vi "UI Event Handler.vi"() -> ()   [LabVIEW 2015]
panel:
  in  "Time Check":bool
  out "Iteration":i32
  in  "Stop":bool
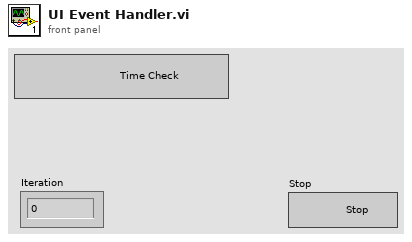
[diagram p1: front panel]
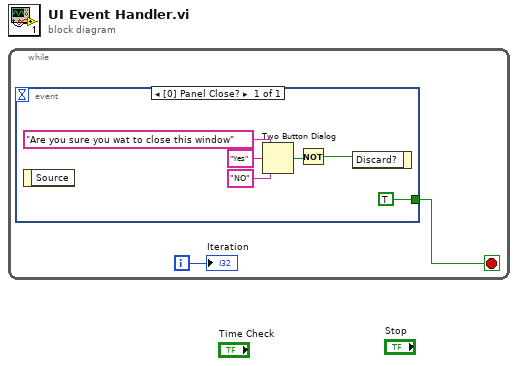
[diagram p0: block diagram]
diagram:
  n1 = while {
    i -> [w2]
    stop <- w1 stop-if-true
    n2 = event shown="[0] Panel Close?" {
      selector: _ -> [_]
      dyn-events: _ -> [_]
      timeout: _ -> [_]
      tunnel: [TRUE] -> w1
      event Panel Close? {
        n3 = event-data() -> ()  [unwired: 1 in, 1 out]
        n4 = Two Button Dialog(message="Are you sure you wat to close this window", 1:"NO" ("F button name (\"Cancel\")"), 2:"Yes" ("T button name (\"OK\")")) -> (T button?=w5:bool)
        n5 = Not(x=w5) -> (.not. x?=w4:bool)
        n6 = event-data("Discard?"=w4) -> ()  [unwired: 1 in, 1 out]
      }
    }
    "Iteration" <- w2
  }
